vi "Navigation Light Control Interface.vi"() -> ()   [LabVIEW 2018]
uses:
  CTL/Yellow Light.ctl
  CTL/Green Light.ctl
  CTL/Red Light.ctl
  CTL/Button.ctl
  CTL/Supply Voltage.ctl
  CTL/Main - SSM - States.ctl
  CTL/FGV - R-W.ctl
panel:
  out "Critical Alert":string="CRITICAL ALERT\n\nBOTH POWER SUPPLIES HAVE FAILED"
  out "S2 InUse":bool
  out "S2 OK":bool
  out "S1 InUse":bool
  out "S1 OK":bool
  out "Supply 1 Voltage":T1 scale=0.0..30.0
  in  "CMD FAULT FLASH":bool
  in  "MBus":bool
  in  "stop":bool
  out "L1 Prime":bool
  out "NL F2":T2
  out "NL E2":T2
  out "NL D2":T2
  out "NL C2":T2
  out "NL B2":T2
  out "NL A2":T2
  out "NL G1":T3
  out "NL H2":T4
  out "?":bool[](array[boolean])
  in  "Config":bool
  in  "Condition ctl":bool
  in  "Test":bool
  out "BUZZER":bool
  in  "Alarms Ack":bool
  in  "NL C":T5
  in  "NL F":T5
  in  "NL H":T5
  in  "NL A":T5
  in  "NL D":T5
  in  "NL E":T5
  in  "NL G":T5
  in  "NL B":T5
  out "NL H1":T4
  out "NL G2":T3
  out "NL F1":T2
  out "NL E1":T2
  out "NL D1":T2
  out "NL C1":T2
  out "NL B1":T2
  out "NL A1":T2
  out "Supply 2 Voltage":T1 scale=0.0..30.0
  # "NAVIGATION LIGHT CONTROL SYSTEM"
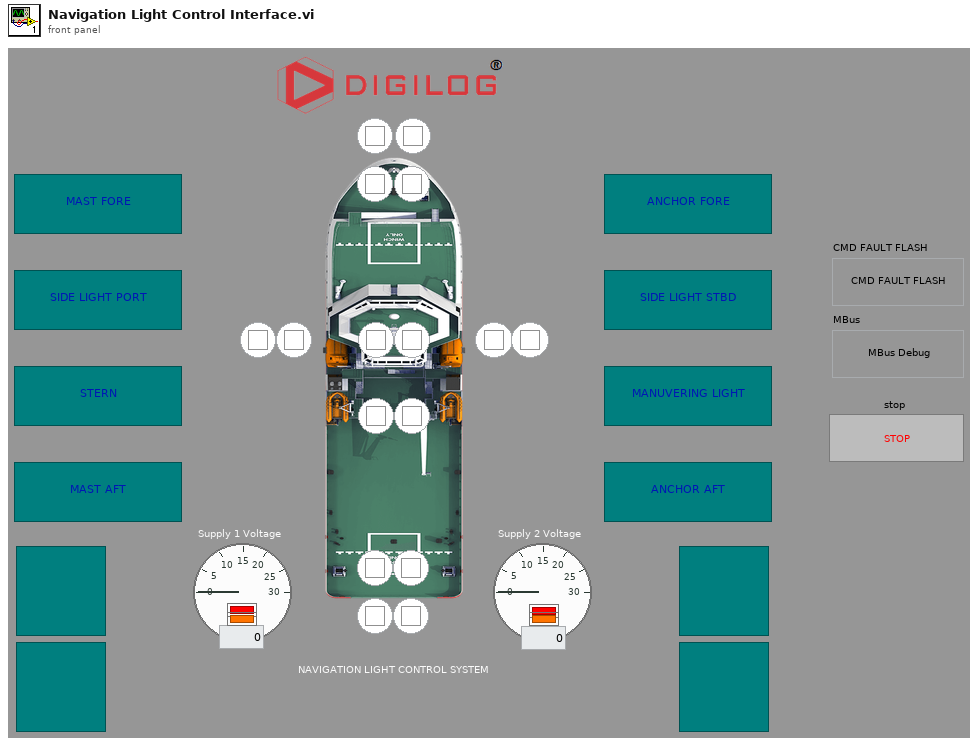
[diagram p1: front panel]
types:
  T1 = typedef "Supply Voltage.ctl" = u32
  T2 = typedef "Yellow Light.ctl" = bool
  T3 = typedef "Green Light.ctl" = bool
  T4 = typedef "Red Light.ctl" = bool
  T5 = typedef "Button.ctl" = bool
  T6 = typedef "Main - SSM - States.ctl" = enum16{"Start", "Read Config", "Event Monitor", "Update Indicators", "Exit"}
  T7 = typedef "FGV - R-W.ctl" = enum16{"W", "R"}
  T8 = enum16{"Lamp A1", "Lamp B1", "Lamp C1", "Lamp D1", "Lamp E1", "Lamp F1", "Lamp G1", "Lamp H1", "Lamp A2", "Lamp B2", "Lamp C2", "Lamp D2", "Lamp E2", "Lamp F2", "Lamp G2", "Lamp H2", "Ack A1", "Ack B1", "Ack C1", "Ack D1", "Ack E1", "Ack F1", "Ack G1", "Ack H1", "Ack A2", "Ack B2", "Ack C2", "Ack D2", "Ack E2", "Ack F2", "Ack G2", "Ack H2", "SSM", "SAS", "LSM", ""}
  T9 = enum8{"Enabled", "Disabled", "Disabled and Grayed Out"}
  T10 = enum32{"Invalid", "Standard", "Closed", "Hidden", "Minimized", "Maximized"}
  T11 = enum16{"Lamp A1", "Lamp B1", "Lamp C1", "Lamp D1", "Lamp E1", "Lamp F1", "Lamp G1", "Lamp H1", "Lamp A2", "Lamp B2", "Lamp C2", "Lamp D2", "Lamp E2", "Lamp F2", "Lamp G2", "Lamp H2", "Ack A1", "Ack B1", "Ack C1", "Ack D1", "Ack E1", "Ack F1", "Ack G1", "Ack H1", "Ack A2", "Ack B2", "Ack C2", "Ack D2", "Ack E2", "Ack F2", "Ack G2", "Ack H2", "SSM", "SAS", "LSM", ""}[]
  T12 = cluster{"Boolean Round":bool, "code":i32, "source":string}
  T13 = typedef "Tags.ctl" = enum16{"Lamp A1", "Lamp B1", "Lamp C1", "Lamp D1", "Lamp E1", "Lamp F1", "Lamp G1", "Lamp H1", "Lamp A2", "Lamp B2", "Lamp C2", "Lamp D2", "Lamp E2", "Lamp F2", "Lamp G2", "Lamp H2", "Ack A1", "Ack B1", "Ack C1", "Ack D1", "Ack E1", "Ack F1", "Ack G1", "Ack H1", "Ack A2", "Ack B2", "Ack C2", "Ack D2", "Ack E2", "Ack F2", "Ack G2", "Ack H2", "SSM", "SAS", "LSM", ""}
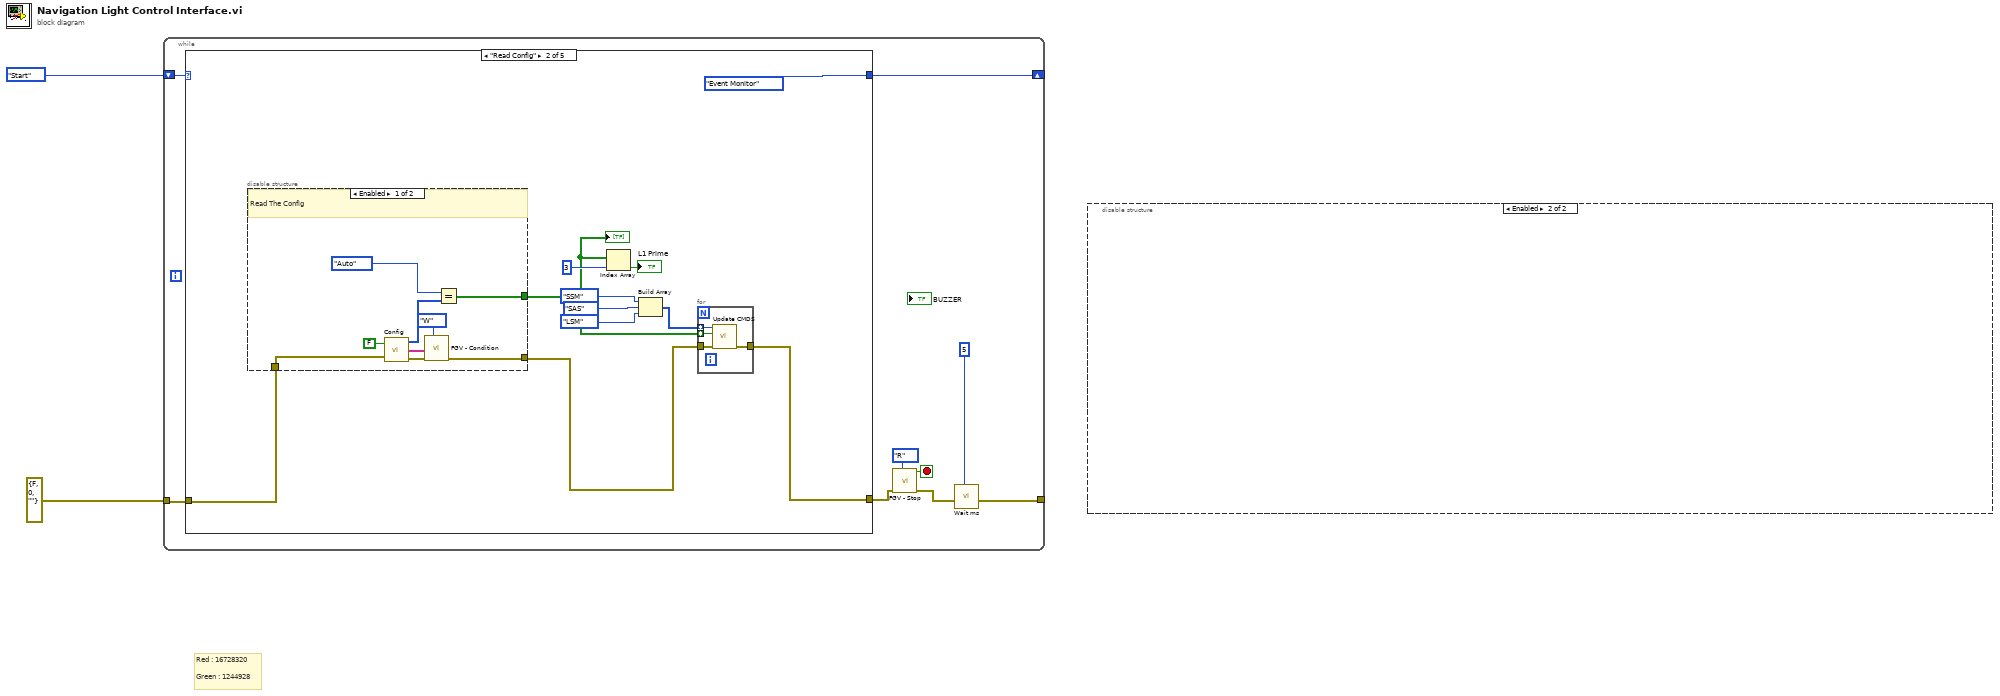
[diagram p0: block diagram]
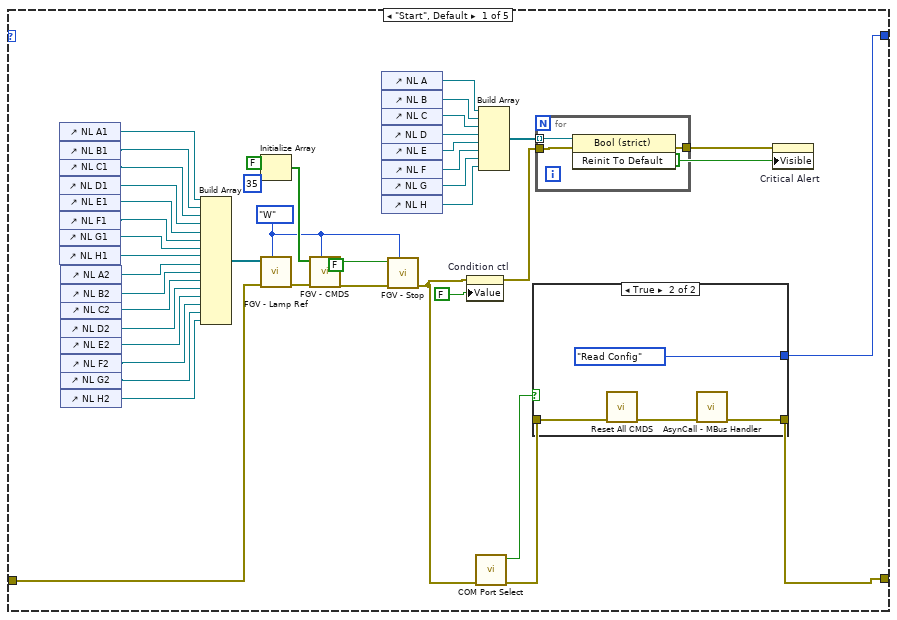
[diagram p3: hidden frame]
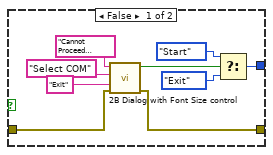
[diagram p4: hidden frame]
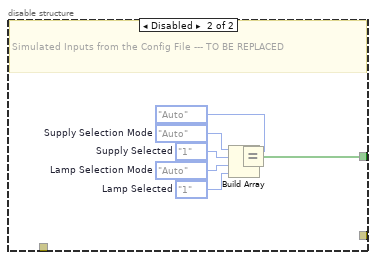
[diagram p5: hidden frame]
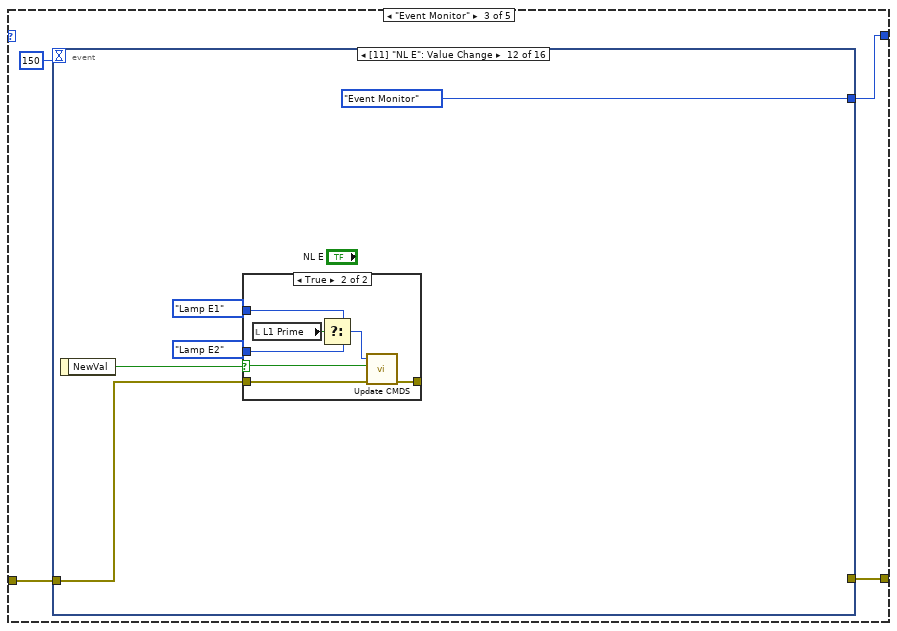
[diagram p6: hidden frame]
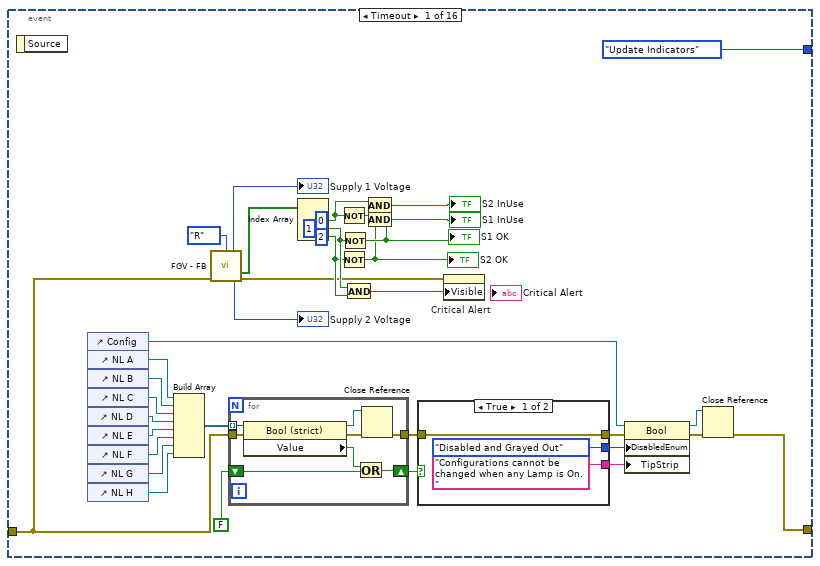
[diagram p7: hidden frame]
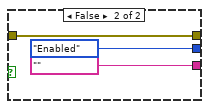
[diagram p8: hidden frame]
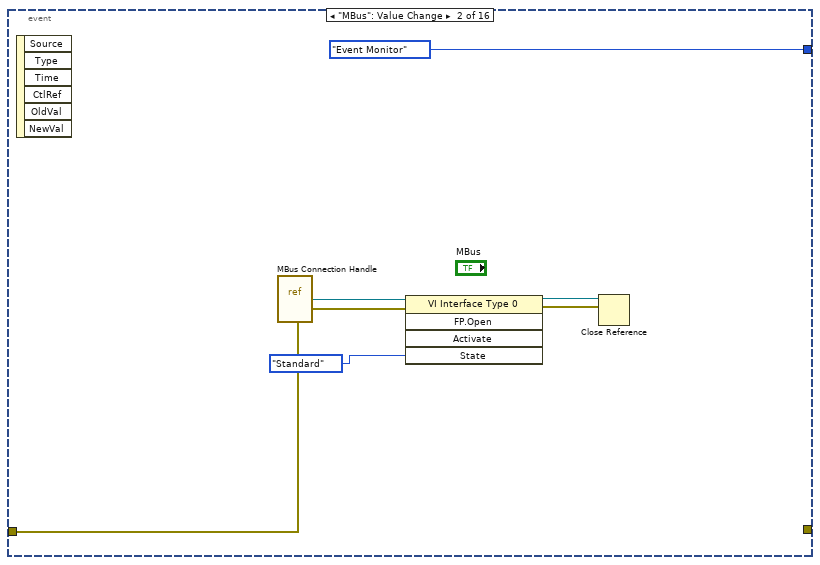
[diagram p9: hidden frame]
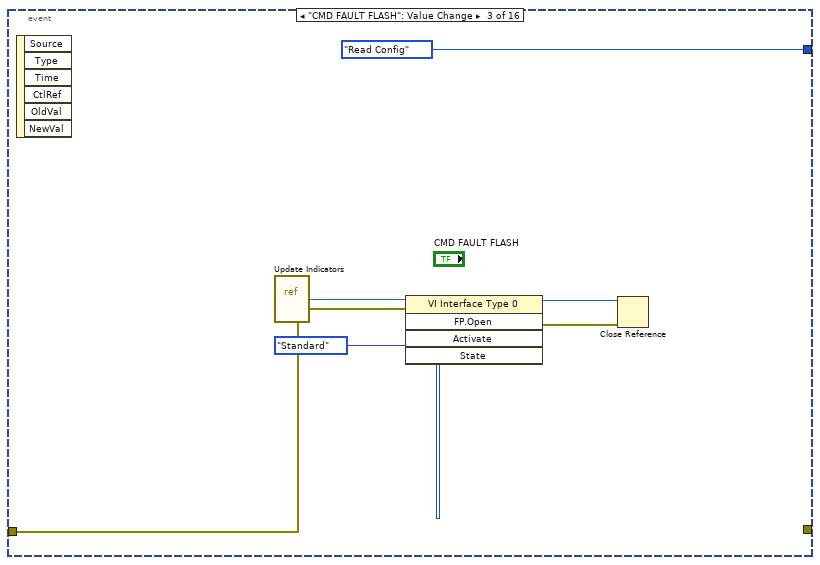
[diagram p10: hidden frame]
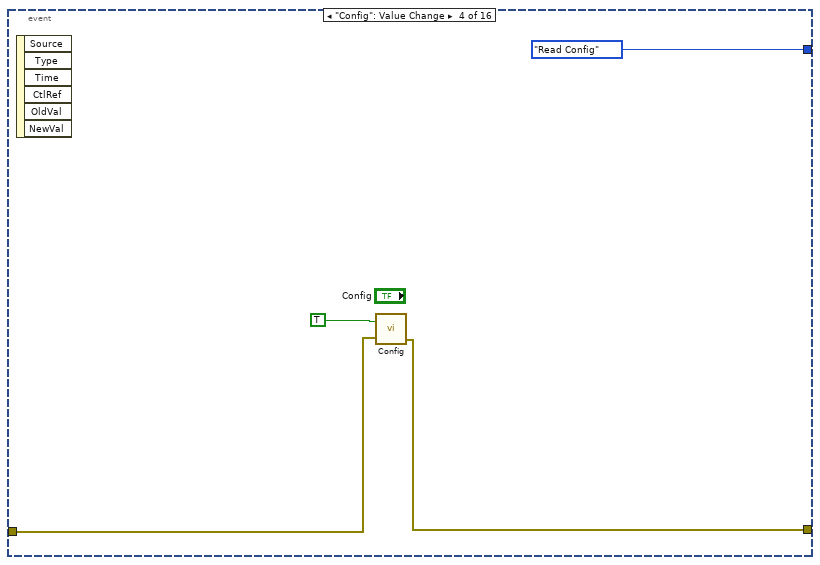
[diagram p11: hidden frame]
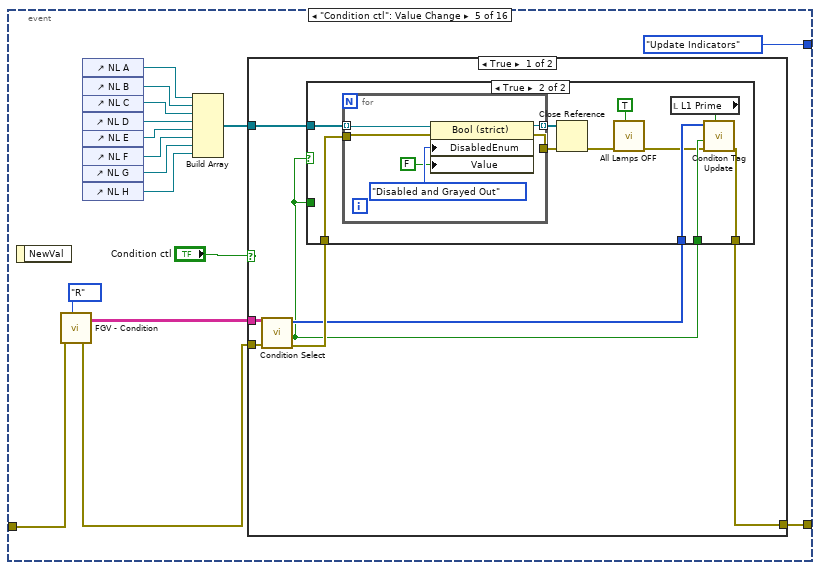
[diagram p12: hidden frame]
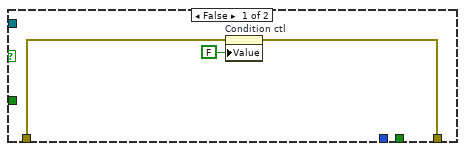
[diagram p13: hidden frame]
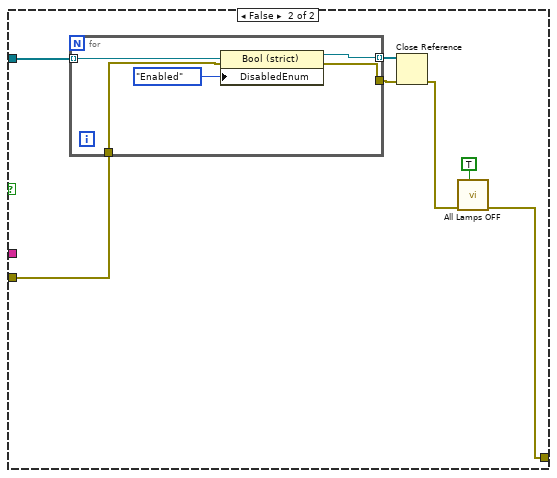
[diagram p14: hidden frame]
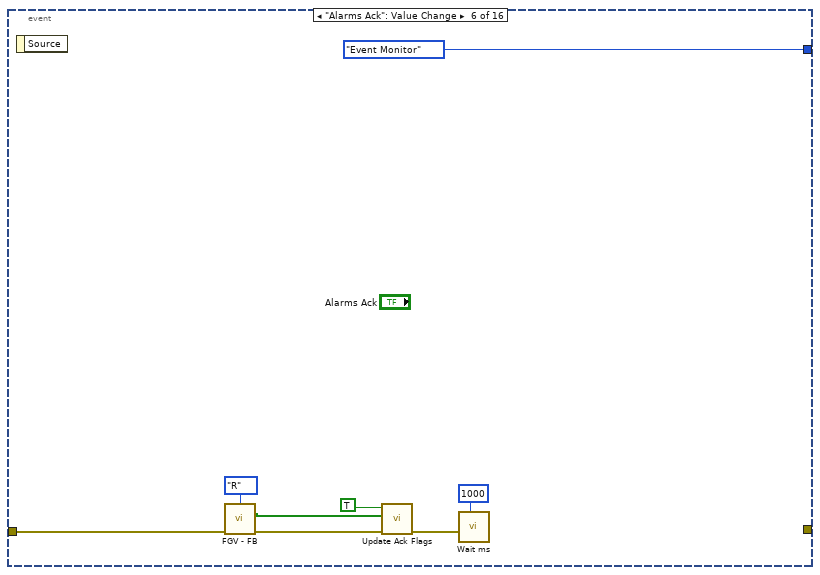
[diagram p15: hidden frame]
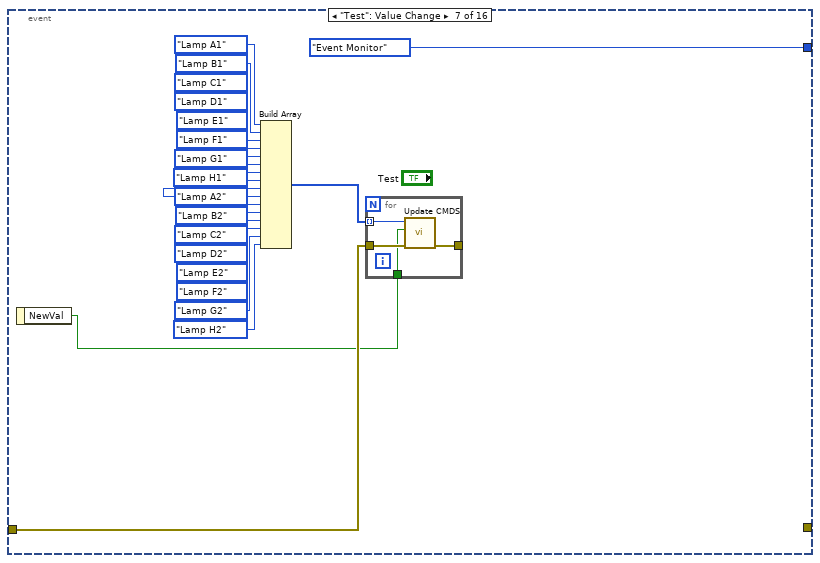
[diagram p16: hidden frame]
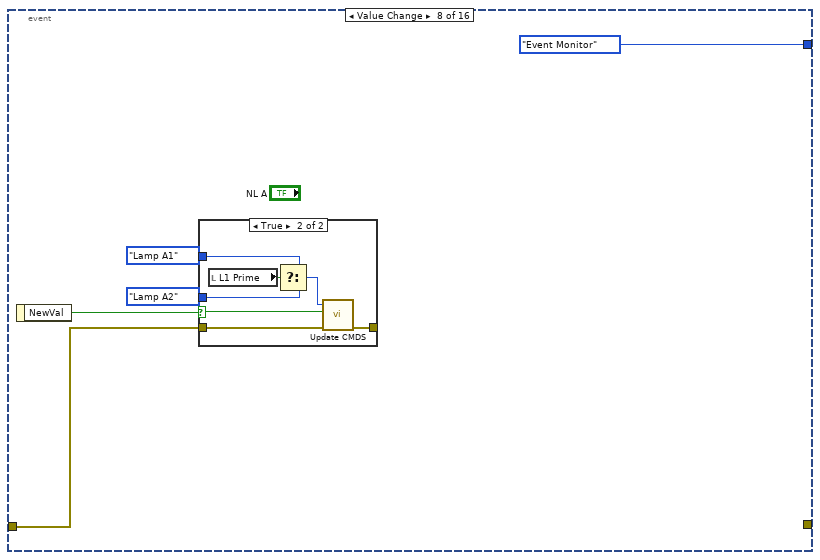
[diagram p17: hidden frame]
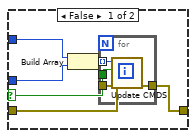
[diagram p18: hidden frame]
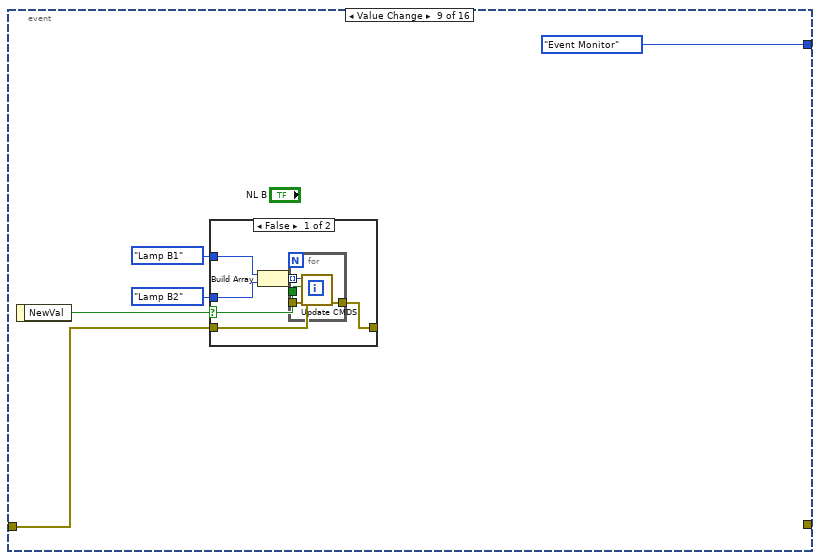
[diagram p19: hidden frame]
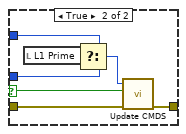
[diagram p20: hidden frame]
diagram:
  # "Red : 16728320\n\nGreen : 1244928"
  n1 = while {
    tunnel: errorcluster {"status"=FALSE, "code"=0, "source"=""} ("error in (no error)") -> [w10]
    shift-right: [w9] -> _
    shift-left: Main_-_SSM_-_States."Start" -> [w11]
    tunnel: [w4] -> _
    stop <- w7 stop-if-true
    n2 = case shown="\"Read Config\"" w11 {
      tunnel: w10 -> [w51 w77 w103 w440 w446]
      tunnel: [w52 Main_-_SSM_-_States."Event Monitor" w105 Main_-_SSM_-_States."Event Monitor" Main_-_SSM_-_States."Exit"] -> w9
      tunnel: [w17 w71 w104 w439 w442] -> w3
      frame "Start", Default {
        w12 = FGV_-_R-W."W" ("Action")
        n3 = control-ref of="NL A1"() -> (w45:refnum<vi>)
        n4 = control-ref of="NL B1"() -> (w43:refnum<vi>)
        n5 = control-ref of="NL C1"() -> (w41:refnum<vi>)
        n6 = control-ref of="NL D1"() -> (w40:refnum<vi>)
        n7 = control-ref of="NL E1"() -> (w37:refnum<vi>)
        n8 = control-ref of="NL F1"() -> (w36:refnum<vi>)
        n9 = control-ref of="NL G1"() -> (w35:refnum<vi>)
        n10 = control-ref of="NL H1"() -> (w34:refnum<vi>)
        n11 = control-ref of="NL A2"() -> (w44:refnum<vi>)
        n12 = control-ref of="NL B2"() -> (w42:refnum<vi>)
        n13 = control-ref of="NL C2"() -> (w39:refnum<vi>)
        n14 = control-ref of="NL D2"() -> (w38:refnum<vi>)
        n15 = control-ref of="NL E2"() -> (w33:refnum<vi>)
        n16 = control-ref of="NL F2"() -> (w32:refnum<vi>)
        n17 = control-ref of="NL G2"() -> (w31:refnum<vi>)
        n18 = control-ref of="NL H2"() -> (w30:refnum<vi>)
        n19 = Build Array(w45, w43, w41, w40, w37, w36, w35, w34, w44, w42, w39, w38, w33, w32, w31, w30) -> (w29:refnum<vi>[])
        n20 = Initialize Array(FALSE ("Acquire? In"), 35 ("dimension size")) -> (w46:bool[])
        n21 = call "FGV - Lamp Ref.vi"("Action"=w12, "error in (no error)"=w51, "Lamp Ref In"=w29) -> ("error out"=w49:errorcluster)  [unwired: 7 in, 1 out]
        n22 = call "FGV - CMDS.vi"("Action"=w12, "error in (no error)"=w49, "Cmd In"=w46) -> ("error out"=w48:errorcluster)  [unwired: 7 in, 1 out]
        n23 = control-ref of="NL A"() -> (w20:refnum<vi>)
        n24 = control-ref of="NL B"() -> (w21:refnum<vi>)
        n25 = control-ref of="NL C"() -> (w22:refnum<vi>)
        n26 = control-ref of="NL D"() -> (w23:refnum<vi>)
        n27 = control-ref of="NL E"() -> (w24:refnum<vi>)
        n28 = control-ref of="NL F"() -> (w25:refnum<vi>)
        n29 = control-ref of="NL G"() -> (w26:refnum<vi>)
        n30 = control-ref of="NL H"() -> (w27:refnum<vi>)
        n31 = call "FGV - Stop.vi"("Action"=w12, "error in (no error)"=w48, "Acquire? In"=FALSE) -> ("error out"=w15:errorcluster)  [unwired: 7 in, 1 out]
        n32 = property on="Condition ctl" class="Bool (strict)"(error in=w15, "Value"=FALSE ("Condition ctl")) -> (error out=w14:errorcluster)  [unwired: 1 in, 1 out]
        n33 = call "COM Port Select.vi"("error in (no error)"=w15) -> ("error out"=w54:errorcluster, "OK"=w53:bool)  [unwired: 9 in]
        n34 = Build Array(w20, w21, w22, w23, w24, w25, w26, w27) -> (w28:refnum<vi>[])
        n35 = case shown="True" w53 {
          tunnel: w54 -> [w63 w68]
          tunnel: [w59 w70] -> w17
          tunnel: [w58 Main_-_SSM_-_States."Read Config"] -> w52
          frame False {
            n36 = call "2B Dialog with Font Size control.vi"("error in (no error)"=w63, "F Button Name (\"Cancel\")"="Exit" ("F Button Name (\"Cancel\")"), "T Button Name (\"OK\")"="Select COM" ("T Button Name (\"OK\")"), "message"="Cannot Proceed Without COM Port") -> ("error out"=w59:errorcluster, "OK"=w61:bool)  [unwired: 6 in]
            n37 = Select(t=Main_-_SSM_-_States."Start", s=w61, f=Main_-_SSM_-_States."Exit") -> (s? t:f=w58:T6)
          }
          frame True {
            n38 = call "Reset All CMDS.vi"("error in (no error)"=w68) -> ("error out"=w67:errorcluster)  [unwired: 10 in]
            n39 = call "AsynCall - MBus Handler.vi"("error in (no error)"=w67) -> ("error out"=w70:errorcluster)  [unwired: 10 in]
          }
        }
        n40 = for {
          tunnel: w28 -> [w57] mode=indexing
          tunnel: w14 -> [w56]
          tunnel: [w55] -> w19
          n41 = invoke class="Bool (strict)" method="Reinit To Default"(reference=w57, error in=w56) -> (error out=w55:errorcluster)  [unwired: 1 in, 2 out]
        }
        n42 = property on="Critical Alert" class="Str"(error in=w19, "Visible"=FALSE) -> ()  [unwired: 1 in, 2 out]
      }
      frame "Read Config" {
        n43 = disable-structure shown="Enabled" {
          disable-tunnel: [w88 w92] -> w74
          disable-tunnel: w77 -> [w86 w91]
          disable-tunnel: [w85 _] -> w72
          frame Enabled {
            # "Read The Config"
            n44 = call "Config.vi"("User Trigger"=FALSE, "error in"=w86) -> ("Config"=w89:u32[], "All Config Data"=w82:string[][], "error out"=w84:errorcluster)
            n45 = call "FGV - Condition.vi"("Action"=FGV_-_R-W."W", "error in (no error)"=w84, "array in"=w82) -> ("error out"=w85:errorcluster)  [unwired: 7 in, 1 out]
            n46 = Equal?(x=enum16{"Auto", "Manual"}."Auto" ("Lamp Selection Mode"), y=w89) -> (x = y?=w88:bool[])
          }
          frame Disabled {
            w96 = enum16{"1", "2"}."1"  # Supply Selected
            w98 = enum16{"1", "2"}."1"  # Lamp Selected
            w93 = enum16{"Manual", "Auto"}."Auto"  # Supply Selection Mode
            w97 = enum16{"Manual", "Auto"}."Auto"  # Lamp Selection Mode
            # "Simulated Inputs from the Config File --- TO BE REPLACED"
            n47 = Build Array(w93, w96, w97, w98) -> (w94:u16[])
            n48 = Equal?(x=enum16{"Auto", "Manual"}."Auto" ("Lamp Selection Mode"), y=w94) -> (x = y?=w92:bool[])
          }
        }
        "?" <- w74
        n49 = Index Array(array=w74, index=3) -> (element=→"L1 Prime":bool)
        n50 = Build Array(T8."SSM" ("Tag"), T8."SAS" ("Tag"), T8."LSM" ("Tag")) -> (w81:T11)
        n51 = for {
          tunnel: w74 -> [w102] mode=indexing
          tunnel: w81 -> [w101] mode=indexing
          tunnel: w72 -> [w100]
          tunnel: [w99] -> w71
          n52 = call "Update CMDS.vi"("error in (no error)"=w100, "New Value"=w102, "Tag"=w101) -> ("error out"=w99:errorcluster)  [unwired: 8 in]
        }
      }
      frame "Event Monitor" {
        n53 = event shown="[11] \"NL E\": Value Change" {
          selector: _ -> [_ _ _ _ _ _ _ _ _ _ _ _ _ _ _ _]
          dyn-events: _ -> [_ _ _ _ _ _ _ _ _ _ _ _ _ _ _ _]
          timeout: 150 -> [_ _ _ _ _ _ _ _ _ _ _ _ _ _ _ _]
          tunnel: w103 -> [w108 w161 w166 w172 w180 w232 w239 w265 w287 w309 w331 w353 w375 w397 w419 _]
          tunnel: [Main_-_SSM_-_States."Update Indicators" Main_-_SSM_-_States."Event Monitor" Main_-_SSM_-_States."Read Config" Main_-_SSM_-_States."Read Config" Main_-_SSM_-_States."Update Indicators" Main_-_SSM_-_States."Event Monitor" Main_-_SSM_-_States."Event Monitor" Main_-_SSM_-_States."Event Monitor" Main_-_SSM_-_States."Event Monitor" Main_-_SSM_-_States."Event Monitor" Main_-_SSM_-_States."Event Monitor" Main_-_SSM_-_States."Event Monitor" Main_-_SSM_-_States."Event Monitor" Main_-_SSM_-_States."Event Monitor" Main_-_SSM_-_States."Event Monitor" Main_-_SSM_-_States."Exit"] -> w105
          tunnel: [w107 _ _ w171 w176 _ _ _ _ _ _ _ _ _ _ _] -> w104
          event Timeout {
            n54 = event-data() -> ()  [unwired: 1 in, 1 out]
            n55 = control-ref of="Config"() -> (w121:refnum<vi>)
            n56 = control-ref of="NL A"() -> (w109:refnum<vi>)
            n57 = control-ref of="NL B"() -> (w110:refnum<vi>)
            n58 = control-ref of="NL C"() -> (w111:refnum<vi>)
            n59 = control-ref of="NL D"() -> (w112:refnum<vi>)
            n60 = control-ref of="NL E"() -> (w113:refnum<vi>)
            n61 = control-ref of="NL F"() -> (w114:refnum<vi>)
            n62 = control-ref of="NL G"() -> (w115:refnum<vi>)
            n63 = control-ref of="NL H"() -> (w116:refnum<vi>)
            n64 = Build Array(w109, w110, w111, w112, w113, w114, w115, w116) -> (w117:refnum<vi>[])
            n65 = call "FGV - FB.vi"("Action"=FGV_-_R-W."R", "error in (no error)"=w108) -> ("Supply 1 Voltage"=→"Supply 1 Voltage":u32, "System FB"=w140:bool[], "Supply 2 Voltage"=→"Supply 2 Voltage":u32, "error out"=w127:errorcluster)  [unwired: 7 in, 3 out]
            n66 = for {
              tunnel: w117 -> [w158] mode=indexing
              shift-right: [w155] -> w118
              shift-left: T5 FALSE ("Value") -> [w153]
              tunnel: [w152] -> w119
              tunnel: w108 -> [w151]
              n67 = property class="Bool (strict)"(reference=w158, error in=w151) -> (reference out=w156:refnum<vi>, error out=w157:errorcluster, "Value"=w154:T5)
              n68 = Or(x=w154, y=w153) -> (x .or. y?=w155:T5)
              n69 = Close Reference(reference=w156, error in (no error)=w157) -> (error out=w152:errorcluster)
            }
            n70 = Index Array(array=w140, index #1=0 ("index"), index #2=1 ("index"), index #3=2 ("index")) -> (element #1=w134:bool, element #2=w130:bool, element #3=w129:bool)
            n71 = Not(x=w134) -> (.not. x?=w131:bool)
            n72 = Not(x=w129) -> (.not. x?=w135:bool)
            "S2 OK" <- w135
            n73 = Not(x=w130) -> (.not. x?=w136:bool)
            "S1 OK" <- w136
            n74 = And(x=w130, y=w129) -> (x .and. y?=w128:bool)
            n75 = And(x=w134, y=w135) -> (x .and. y?=→"S2 InUse":bool)
            n76 = And(x=w131, y=w136) -> (x .and. y?=→"S1 InUse":bool)
            n77 = case shown="True" w118 {
              tunnel: w119 -> [w147 w150]
              tunnel: [w147 w150] -> w123
              tunnel: ["Configurations cannot be changed when any Lamp is On. " ("Tip Strip") "" ("Tip Strip")] -> w124
              tunnel: [T9."Disabled and Grayed Out" ("Disabled") T9."Enabled" ("Disabled")] -> w125
              frame True {
              }
              frame False {
              }
            }
            n78 = property on="Critical Alert" class="Str"(error in=w127, "Visible"=w128) -> ()  [unwired: 1 in, 2 out]
            n79 = property class="Bool"(reference=w121, error in=w123, "DisabledEnum"=w125, "TipStrip"=w124) -> (reference out=w126:refnum<vi>, error out=w122:errorcluster)
            n80 = Close Reference(reference=w126, error in (no error)=w122) -> (error out=w107:errorcluster)
          }
          event "MBus": Value Change {
            n81 = event-data() -> ()  [unwired: 1 in, 6 out]
            n82 = vi-ref "MBus Connection Handle.vi"() -> (w162:refnum<vi>)
            n83 = invoke class="VI Interface Type 0" method="FP.Open"(reference=w162, error in=w161, "State"=T10."Standard") -> (reference out=w163:refnum<vi>, error out=w164:errorcluster)  [unwired: 2 in, 3 out]
            n84 = Close Reference(reference=w163, error in (no error)=w164) -> ()  [unwired: 1 out]
          }
          event "CMD FAULT FLASH": Value Change {
            n85 = event-data() -> ()  [unwired: 1 in, 6 out]
            n86 = vi-ref "Update Indicators.vi"() -> (w167:refnum<vi>)
            n87 = invoke class="VI Interface Type 0" method="FP.Open"(reference=w167, error in=w166, "State"=T10."Standard") -> (reference out=w169:refnum<vi>, error out=w170:errorcluster)  [unwired: 2 in, 3 out]
            n88 = Close Reference(reference=w169, error in (no error)=w170) -> ()  [unwired: 1 out]
          }
          event "Config": Value Change {
            n89 = event-data() -> ()  [unwired: 1 in, 6 out]
            n90 = call "Config.vi"("User Trigger"=TRUE, "error in"=w172) -> ("error out"=w171:errorcluster)  [unwired: 2 out]
          }
          event "Condition ctl": Value Change {
            n91 = event-data() -> ()  [unwired: 1 in, 1 out]
            n92 = call "FGV - Condition.vi"("Action"=FGV_-_R-W."R", "error in (no error)"=w180) -> ("error out"=w178:errorcluster, "array out"=w177:string[][])  [unwired: 8 in]
            n93 = control-ref of="NL A"() -> (w182:refnum<vi>)
            n94 = control-ref of="NL B"() -> (w183:refnum<vi>)
            n95 = control-ref of="NL C"() -> (w184:refnum<vi>)
            n96 = control-ref of="NL D"() -> (w185:refnum<vi>)
            n97 = control-ref of="NL E"() -> (w186:refnum<vi>)
            n98 = control-ref of="NL F"() -> (w187:refnum<vi>)
            n99 = control-ref of="NL G"() -> (w188:refnum<vi>)
            n100 = control-ref of="NL H"() -> (w189:refnum<vi>)
            n101 = Build Array(w182, w183, w184, w185, w186, w187, w188, w189) -> (w190:refnum<vi>[])
            n102 = case shown="True" "Condition ctl" {
              tunnel: w190 -> [w197 w222]
              tunnel: w178 -> [w196 w219]
              tunnel: w177 -> [w195 _]
              tunnel: [w192 w220] -> w176
              frame True {
                n103 = call "Condition Select.vi"("error in (no error)"=w196, "array in"=w195) -> ("error out"=w194:T12, "OK?"=w191:bool, "Array"=w193:T13[])  [unwired: 6 in, 1 out]
                n104 = case shown="True" w191 {
                  tunnel: w197 -> [_ w209]
                  tunnel: w194 -> [w200 w208]
                  tunnel: w191 -> [_ _]
                  tunnel: w193 -> [_ w206]
                  tunnel: [w199 w205] -> w192
                  tunnel: w191 -> [_ w204]
                  frame False {
                    n105 = property on="Condition ctl" class="Bool (strict)"(error in=w200, "Value"=FALSE ("Condition ctl")) -> (error out=w199:errorcluster)  [unwired: 1 in, 1 out]
                  }
                  frame True {
                    n106 = for {
                      tunnel: w209 -> [w217] mode=indexing
                      tunnel: [w216] -> w210 mode=indexing
                      tunnel: [w215] -> w211
                      tunnel: w208 -> [w213]
                      n107 = property class="Bool (strict)"(reference=w217, error in=w213, "DisabledEnum"=T9."Disabled and Grayed Out" ("Disabled"), "Value"=FALSE) -> (reference out=w216:refnum<vi>, error out=w215:errorcluster)
                    }
                    n108 = Close Reference(reference=w210, error in (no error)=w211) -> (error out=w202:errorcluster)
                    n109 = call "All Lamps OFF.vi"("L1 Prime"=TRUE, "error in (no error)"=w202) -> ("error out"=w201:T12)  [unwired: 9 in]
                    n110 = local read "L1 Prime"() -> (w207:bool)
                    n111 = call "Conditon Tag Update.vi"("L1 Prime"=w207, "error in (no error)"=w201, "OK?"=w204, "Array"=w206) -> ("error out"=w205:T12)  [unwired: 7 in]
                  }
                }
              }
              frame False {
                n112 = for {
                  tunnel: w222 -> [w229] mode=indexing
                  tunnel: [w228] -> w223 mode=indexing
                  tunnel: [w227] -> w224
                  tunnel: w219 -> [w225]
                  n113 = property class="Bool (strict)"(reference=w229, error in=w225, "DisabledEnum"=T9."Enabled" ("Disabled")) -> (reference out=w228:refnum<vi>, error out=w227:errorcluster)
                }
                n114 = Close Reference(reference=w223, error in (no error)=w224) -> (error out=w221:errorcluster)
                n115 = call "All Lamps OFF.vi"("L1 Prime"=TRUE, "error in (no error)"=w221) -> ("error out"=w220:T12)  [unwired: 9 in]
              }
            }
          }
          event "Alarms Ack": Value Change {
            n116 = event-data() -> ()  [unwired: 1 in, 1 out]
            n117 = call "FGV - FB.vi"("Action"=FGV_-_R-W."R", "error in (no error)"=w232) -> ("Fault FB"=w230:bool[], "error out"=w231:errorcluster)  [unwired: 7 in, 5 out]
            n118 = call "Update Ack Flags.vi"("error in (no error)"=w231, "Cmd Value"=w230, "Value"=TRUE) -> ("Error Out"=w234:errorcluster)  [unwired: 8 in]
            n119 = call "Wait ms.vi"("milliseconds to wait"=u32 1000, "error in (no error)"=w234) -> ()  [unwired: 9 in, 1 out]
          }
          event "Test": Value Change {
            n120 = event-data() -> ("NewVal"=w238:bool)  [unwired: 1 in]
            n121 = Build Array(T8."Lamp A1" ("Tag"), T8."Lamp B1" ("Tag"), T8."Lamp C1" ("Tag"), T8."Lamp D1" ("Tag"), T8."Lamp E1" ("Tag"), T8."Lamp F1" ("Tag"), T8."Lamp G1" ("Tag"), T8."Lamp H1" ("Tag"), T8."Lamp A2" ("Tag"), T8."Lamp B2" ("Tag"), T8."Lamp C2" ("Tag"), T8."Lamp D2" ("Tag"), T8."Lamp E2" ("Tag"), T8."Lamp F2" ("Tag"), T8."Lamp G2" ("Tag"), T8."Lamp H2" ("Tag")) -> (w240:T11)
            n122 = for {
              tunnel: w240 -> [w261] mode=indexing
              tunnel: w239 -> [w260]
              tunnel: [w259] -> _
              tunnel: w238 -> [w258]
              n123 = call "Update CMDS.vi"("error in (no error)"=w260, "New Value"=w258, "Tag"=w261) -> ("error out"=w259:errorcluster)  [unwired: 8 in]
            }
          }
          event Value Change {
            n124 = event-data() -> ("NewVal"=w266:T5)  [unwired: 1 in]
            n125 = case shown="True" w266 {
              selector: w266 -> [w269 w282]
              tunnel: w265 -> [w271 w280]
              tunnel: [w270 w279] -> _
              tunnel: T8."Lamp A2" ("Tag") -> [w268 w278]
              tunnel: T8."Lamp A1" ("Tag") -> [w267 w277]
              frame False {
                n126 = Build Array(w267, w268) -> (w272:T11)
                n127 = for {
                  tunnel: w272 -> [w276] mode=indexing
                  tunnel: w271 -> [w275]
                  tunnel: [w274] -> w270
                  tunnel: w269 -> [w273]
                  n128 = call "Update CMDS.vi"("error in (no error)"=w275, "New Value"=w273, "Tag"=w276) -> ("error out"=w274:errorcluster)  [unwired: 8 in]
                }
              }
              frame True {
                n129 = local read "L1 Prime"() -> (w283:bool)
                n130 = Select(t=w277, s=w283, f=w278) -> (s? t:f=w281:T8)
                n131 = call "Update CMDS.vi"("error in (no error)"=w280, "New Value"=w282, "Tag"=w281) -> ("error out"=w279:errorcluster)  [unwired: 8 in]
              }
            }
          }
          event Value Change {
            n132 = event-data() -> ("NewVal"=w288:T5)  [unwired: 1 in]
            n133 = case shown="False" w288 {
              selector: w288 -> [w291 w304]
              tunnel: w287 -> [w293 w302]
              tunnel: [w292 w301] -> _
              tunnel: T8."Lamp B2" ("Tag") -> [w290 w300]
              tunnel: T8."Lamp B1" ("Tag") -> [w289 w299]
              frame False {
                n134 = Build Array(w289, w290) -> (w294:T11)
                n135 = for {
                  tunnel: w294 -> [w298] mode=indexing
                  tunnel: w293 -> [w297]
                  tunnel: [w296] -> w292
                  tunnel: w291 -> [w295]
                  n136 = call "Update CMDS.vi"("error in (no error)"=w297, "New Value"=w295, "Tag"=w298) -> ("error out"=w296:errorcluster)  [unwired: 8 in]
                }
              }
              frame True {
                n137 = local read "L1 Prime"() -> (w305:bool)
                n138 = Select(t=w299, s=w305, f=w300) -> (s? t:f=w303:T8)
                n139 = call "Update CMDS.vi"("error in (no error)"=w302, "New Value"=w304, "Tag"=w303) -> ("error out"=w301:errorcluster)  [unwired: 8 in]
              }
            }
          }
          event Value Change {
            n140 = event-data() -> ("NewVal"=w310:T5)  [unwired: 1 in]
            n141 = case shown="False" w310 {
              selector: w310 -> [w313 w326]
              tunnel: w309 -> [w315 w324]
              tunnel: [w314 w323] -> _
              tunnel: T8."Lamp C2" ("Tag") -> [w312 w322]
              tunnel: T8."Lamp C1" ("Tag") -> [w311 w321]
              frame False {
                n142 = Build Array(w311, w312) -> (w316:T11)
                n143 = for {
                  tunnel: w316 -> [w320] mode=indexing
                  tunnel: w315 -> [w319]
                  tunnel: [w318] -> w314
                  tunnel: w313 -> [w317]
                  n144 = call "Update CMDS.vi"("error in (no error)"=w319, "New Value"=w317, "Tag"=w320) -> ("error out"=w318:errorcluster)  [unwired: 8 in]
                }
              }
              frame True {
                n145 = local read "L1 Prime"() -> (w327:bool)
                n146 = Select(t=w321, s=w327, f=w322) -> (s? t:f=w325:T8)
                n147 = call "Update CMDS.vi"("error in (no error)"=w324, "New Value"=w326, "Tag"=w325) -> ("error out"=w323:errorcluster)  [unwired: 8 in]
              }
            }
          }
          event Value Change {
            n148 = event-data() -> ("NewVal"=w332:T5)  [unwired: 1 in]
            n149 = case shown="False" w332 {
              selector: w332 -> [w335 w348]
              tunnel: w331 -> [w337 w346]
              tunnel: [w336 w345] -> _
              tunnel: T8."Lamp D2" ("Tag") -> [w334 w344]
              tunnel: T8."Lamp D1" ("Tag") -> [w333 w343]
              frame False {
                n150 = Build Array(w333, w334) -> (w338:T11)
                n151 = for {
                  tunnel: w338 -> [w342] mode=indexing
                  tunnel: w337 -> [w341]
                  tunnel: [w340] -> w336
                  tunnel: w335 -> [w339]
                  n152 = call "Update CMDS.vi"("error in (no error)"=w341, "New Value"=w339, "Tag"=w342) -> ("error out"=w340:errorcluster)  [unwired: 8 in]
                }
              }
              frame True {
                n153 = local read "L1 Prime"() -> (w349:bool)
                n154 = Select(t=w343, s=w349, f=w344) -> (s? t:f=w347:T8)
                n155 = call "Update CMDS.vi"("error in (no error)"=w346, "New Value"=w348, "Tag"=w347) -> ("error out"=w345:errorcluster)  [unwired: 8 in]
              }
            }
          }
          event Value Change {
            n156 = event-data() -> ("NewVal"=w354:T5)  [unwired: 1 in]
            n157 = case shown="True" w354 {
              selector: w354 -> [w357 w370]
              tunnel: w353 -> [w359 w368]
              tunnel: [w358 w367] -> _
              tunnel: T8."Lamp E2" ("Tag") -> [w356 w366]
              tunnel: T8."Lamp E1" ("Tag") -> [w355 w365]
              frame False {
                n158 = Build Array(w355, w356) -> (w360:T11)
                n159 = for {
                  tunnel: w360 -> [w364] mode=indexing
                  tunnel: w359 -> [w363]
                  tunnel: [w362] -> w358
                  tunnel: w357 -> [w361]
                  n160 = call "Update CMDS.vi"("error in (no error)"=w363, "New Value"=w361, "Tag"=w364) -> ("error out"=w362:errorcluster)  [unwired: 8 in]
                }
              }
              frame True {
                n161 = local read "L1 Prime"() -> (w371:bool)
                n162 = Select(t=w365, s=w371, f=w366) -> (s? t:f=w369:T8)
                n163 = call "Update CMDS.vi"("error in (no error)"=w368, "New Value"=w370, "Tag"=w369) -> ("error out"=w367:errorcluster)  [unwired: 8 in]
              }
            }
          }
          event Value Change {
            n164 = event-data() -> ("NewVal"=w376:T5)  [unwired: 1 in]
            n165 = case shown="True" w376 {
              selector: w376 -> [w379 w392]
              tunnel: w375 -> [w381 w390]
              tunnel: [w380 w389] -> _
              tunnel: T8."Lamp F2" ("Tag") -> [w378 w388]
              tunnel: T8."Lamp F1" ("Tag") -> [w377 w387]
              frame False {
                n166 = Build Array(w377, w378) -> (w382:T11)
                n167 = for {
                  tunnel: w382 -> [w386] mode=indexing
                  tunnel: w381 -> [w385]
                  tunnel: [w384] -> w380
                  tunnel: w379 -> [w383]
                  n168 = call "Update CMDS.vi"("error in (no error)"=w385, "New Value"=w383, "Tag"=w386) -> ("error out"=w384:errorcluster)  [unwired: 8 in]
                }
              }
              frame True {
                n169 = local read "L1 Prime"() -> (w393:bool)
                n170 = Select(t=w387, s=w393, f=w388) -> (s? t:f=w391:T8)
                n171 = call "Update CMDS.vi"("error in (no error)"=w390, "New Value"=w392, "Tag"=w391) -> ("error out"=w389:errorcluster)  [unwired: 8 in]
              }
            }
          }
          event Value Change {
            n172 = event-data() -> ("NewVal"=w398:T5)  [unwired: 1 in]
            n173 = case shown="True" w398 {
              selector: w398 -> [w401 w414]
              tunnel: w397 -> [w403 w412]
              tunnel: [w402 w411] -> _
              tunnel: T8."Lamp G2" ("Tag") -> [w400 w410]
              tunnel: T8."Lamp G1" ("Tag") -> [w399 w409]
              frame False {
                n174 = Build Array(w399, w400) -> (w404:T11)
                n175 = for {
                  tunnel: w404 -> [w408] mode=indexing
                  tunnel: w403 -> [w407]
                  tunnel: [w406] -> w402
                  tunnel: w401 -> [w405]
                  n176 = call "Update CMDS.vi"("error in (no error)"=w407, "New Value"=w405, "Tag"=w408) -> ("error out"=w406:errorcluster)  [unwired: 8 in]
                }
              }
              frame True {
                n177 = local read "L1 Prime"() -> (w415:bool)
                n178 = Select(t=w409, s=w415, f=w410) -> (s? t:f=w413:T8)
                n179 = call "Update CMDS.vi"("error in (no error)"=w412, "New Value"=w414, "Tag"=w413) -> ("error out"=w411:errorcluster)  [unwired: 8 in]
              }
            }
          }
          event Value Change {
            n180 = event-data() -> ("NewVal"=w420:T5)  [unwired: 1 in]
            n181 = case shown="True" w420 {
              selector: w420 -> [w423 w436]
              tunnel: w419 -> [w425 w434]
              tunnel: [w424 w433] -> _
              tunnel: T8."Lamp H2" ("Tag") -> [w422 w432]
              tunnel: T8."Lamp H1" ("Tag") -> [w421 w431]
              frame False {
                n182 = Build Array(w421, w422) -> (w426:T11)
                n183 = for {
                  tunnel: w426 -> [w430] mode=indexing
                  tunnel: w425 -> [w429]
                  tunnel: [w428] -> w424
                  tunnel: w423 -> [w427]
                  n184 = call "Update CMDS.vi"("error in (no error)"=w429, "New Value"=w427, "Tag"=w430) -> ("error out"=w428:errorcluster)  [unwired: 8 in]
                }
              }
              frame True {
                n185 = local read "L1 Prime"() -> (w437:bool)
                n186 = Select(t=w431, s=w437, f=w432) -> (s? t:f=w435:T8)
                n187 = call "Update CMDS.vi"("error in (no error)"=w434, "New Value"=w436, "Tag"=w435) -> ("error out"=w433:errorcluster)  [unwired: 8 in]
              }
            }
          }
          event "stop": Value Change {
            n188 = event-data() -> ()  [unwired: 1 in, 1 out]
          }
        }
      }
      frame "Update Indicators" {
        n189 = call "Update Indicators.vi"("error in (no error)"=w440) -> ("error out"=w439:errorcluster)  [unwired: 10 in]
      }
      frame "Exit" {
        n190 = call "FGV - Stop.vi"("Action"=FGV_-_R-W."W", "error in (no error)"=w446, "Acquire? In"=TRUE) -> ("error out"=w444:errorcluster)  [unwired: 7 in, 1 out]
        n191 = call "Wait ms.vi"("milliseconds to wait"=u32 2500, "error in (no error)"=w444) -> ("error out"=w442:errorcluster)  [unwired: 9 in]
      }
    }
    n192 = call "FGV - Stop.vi"("Action"=FGV_-_R-W."R", "error in (no error)"=w3) -> ("error out"=w5:errorcluster, "Acquire? Out"=w7:bool)  [unwired: 8 in]
    n193 = call "Wait ms.vi"("milliseconds to wait"=u32 5, "error in (no error)"=w5) -> ("error out"=w4:errorcluster)  [unwired: 9 in]
  }
  n194 = disable-structure shown="Enabled" {
    frame Disabled {
    }
    frame Enabled {
    }
  }
